vi "FGVPartA.vi"() -> ()   [LabVIEW 2014]
panel:
  out "count":i32
  in  "stop":bool
  out "NumericOut":i32
  # "Part A"
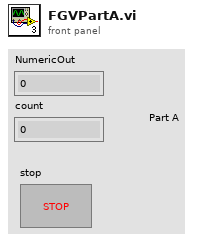
[diagram p1: front panel]
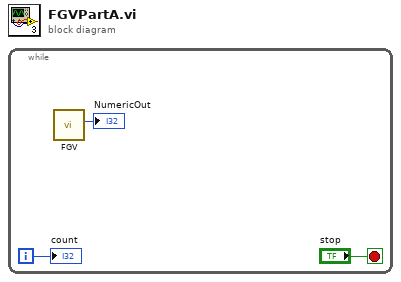
[diagram p0: block diagram]
diagram:
  n1 = while {
    i -> [w1]
    stop <- "stop" stop-if-true
    n2 = call "FGV.vi"() -> ("NumericOut"=→"NumericOut":i32)  [unwired: 11 in]
    "count" <- w1
  }
